vi "Format Section Header.vi"(0 "header":string, 5 "body":string) -> (4 "formatted section header":string)   [LabVIEW 2020]
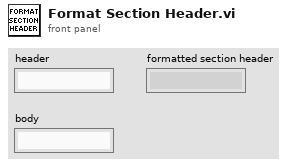
[diagram p1: front panel]
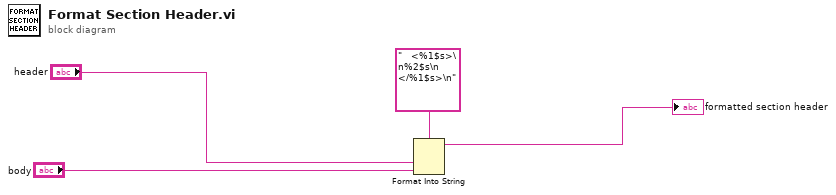
[diagram p0: block diagram]
diagram:
  n1 = Format Into String(format string="   <%1$s>\n%2$s\n   </%1$s>\n", "header", "body") -> (resulting string=→"formatted section header":string)  [unwired: 2 in, 1 out]
